vi "4 probe data v1.2.vi"() -> ()   [LabVIEW 2014]
uses:
  <vilib>/Analysis/baseanly.llb/Mean (DBL).vi
  <vilib>/MakerHub/LINX/Public/Peripherals/Analog/Analog Read 1 Chan.vi
  <instrlib>/Tektronix TDS 200 1000 2000 Series/Tektronix TDS 200 1000 2000 Series.lvlib
  <vilib>/MakerHub/LINX/LMH-LINX.lvlib
  <vilib>/Analysis/NI_AALBase.lvlib
panel:
  in  "Stop Button":bool
  out "Ard 4":dbl
  out "Ard 3":dbl
  out "Ard 2":dbl
  out "Ard 1":dbl
  out "Ard 0":dbl
  out "Data Ch4":string
  in  "Save File Ch4":path=path "C:/Users/Administrator/Documents/Device-characterization-setup/IV-Trace/Data/2015_xx_xx_xxxx_4-probe/2015_xx_xx_xxxx_Ch4_001.txt"
  out "Ard3-Osc4":cluster{"Y":dbl[], "Y":dbl[]}[](graph)
  out "Data Ch3":string
  in  "Save File Ch3":path=path "C:/Users/Administrator/Documents/Device-characterization-setup/IV-Trace/Data/2015_xx_xx_xxxx_4-probe/2015_xx_xx_xxxx_Ch3_001.txt"
  out "Ard2-Osc 3":cluster{"Y":dbl[], "Y":dbl[]}[](graph)
  out "Data Ch2":string
  in  "Save File Ch2":path=path "C:/Users/Administrator/Documents/Device-characterization-setup/IV-Trace/Data/2015_xx_xx_xxxx_4-probe/2015_xx_xx_xxxx_Ch2_001.txt"
  out "Ard1-Osc 2":cluster{"Y":dbl[], "Y":dbl[]}[](graph)
  out "Data Ch1":string
  in  "Save File Ch1":path=path "C:/Users/Administrator/Documents/Device-characterization-setup/IV-Trace/Data/2015_xx_xx_xxxx_4-probe/2015_xx_xx_xxxx_Ch1_001.txt"
  out "Ard0-Osc 1":cluster{"Y":dbl[], "Y":dbl[]}[](graph)
  out "Ch1":dbl
  out "Ch2":dbl
  out "Ch3":dbl
  out "Ch4":dbl
  out "Loop Rate (Hz)":u32
  out "Analog Data 4":dbl(graph)
  in  "AI Channel 4":u8=4
  in  "AI Channel 3":u8=3
  in  "AI Channel 2":u8=2
  in  "AI Channel 1":u8=1
  in  "AI Channel 0":u8
  in  "Serial Port":refnum<visa-resource-name>="COM6"
  in  "Channel 4 (3: Channel 4)":u16(ring)=3 items=["Channel 1", "Channel 2", "Channel 3", "Channel 4", "Math", "Reference A", "Reference B", "Reference C", "Reference D"]
  in  "Probe Attenuation 4 (0.1)":dbl=0.1
  in  "Vertical Coupling 4 (1: DC)":u16(ring)=1 items=["AC", "DC", "Ground"]
  in  "Channel 3 (2: Channel 3)":u16(ring)=2 items=["Channel 1", "Channel 2", "Channel 3", "Channel 4", "Math", "Reference A", "Reference B", "Reference C", "Reference D"]
  in  "Probe Attenuation 3 (0.1)":dbl=0.1
  in  "Vertical Coupling 3 (1: DC)":u16(ring)=1 items=["AC", "DC", "Ground"]
  in  "Channel 2 (1: Channel 2)":u16(ring)=1 items=["Channel 1", "Channel 2", "Channel 3", "Channel 4", "Math", "Reference A", "Reference B", "Reference C", "Reference D"]
  in  "Channel 1 (0: Channel 1)":u16(ring) items=["Channel 1", "Channel 2", "Channel 3", "Channel 4", "Math", "Reference A", "Reference B", "Reference C", "Reference D"]
  in  "Serial Configuration":T1={"Baud Rate"=9600, "Parity"=0, "Stop Bits"=10, "Flow Control"=2} {"Flow Control" items=["None", "XON/XOFF", "RTS/CTS", "XON/XOFF & RTS/CTS", "DTR/DSR", "XON/XOFF & DTR/DSR"]; "Stop Bits" items=["1.0"=10, "1.5"=15, "2.0"=20]; "Parity" items=["None", "Odd", "Even", "Mark", "Space"]; "Baud Rate" items=["300"=300, "600"=600, "1200"=1200, "2400"=2400, "4800"=4800, "9600"=9600, "19200"=19200]}
  in  "Probe Attenuation 2 (0.1)":dbl=0.1
  in  "Vertical Coupling 2 (1: DC)":u16(ring)=1 items=["AC", "DC", "Ground"]
  in  "Probe Attenuation 1 (0.1)":dbl=0.1
  in  "Vertical Coupling 1 (1: DC)":u16(ring)=1 items=["AC", "DC", "Ground"]
  in  "Timeout (10000 ms)":u32=500
  in  "VISA resource name":refnum<visa-resource-name>="USB0::0x0699::0x03A6::C044157::INSTR"
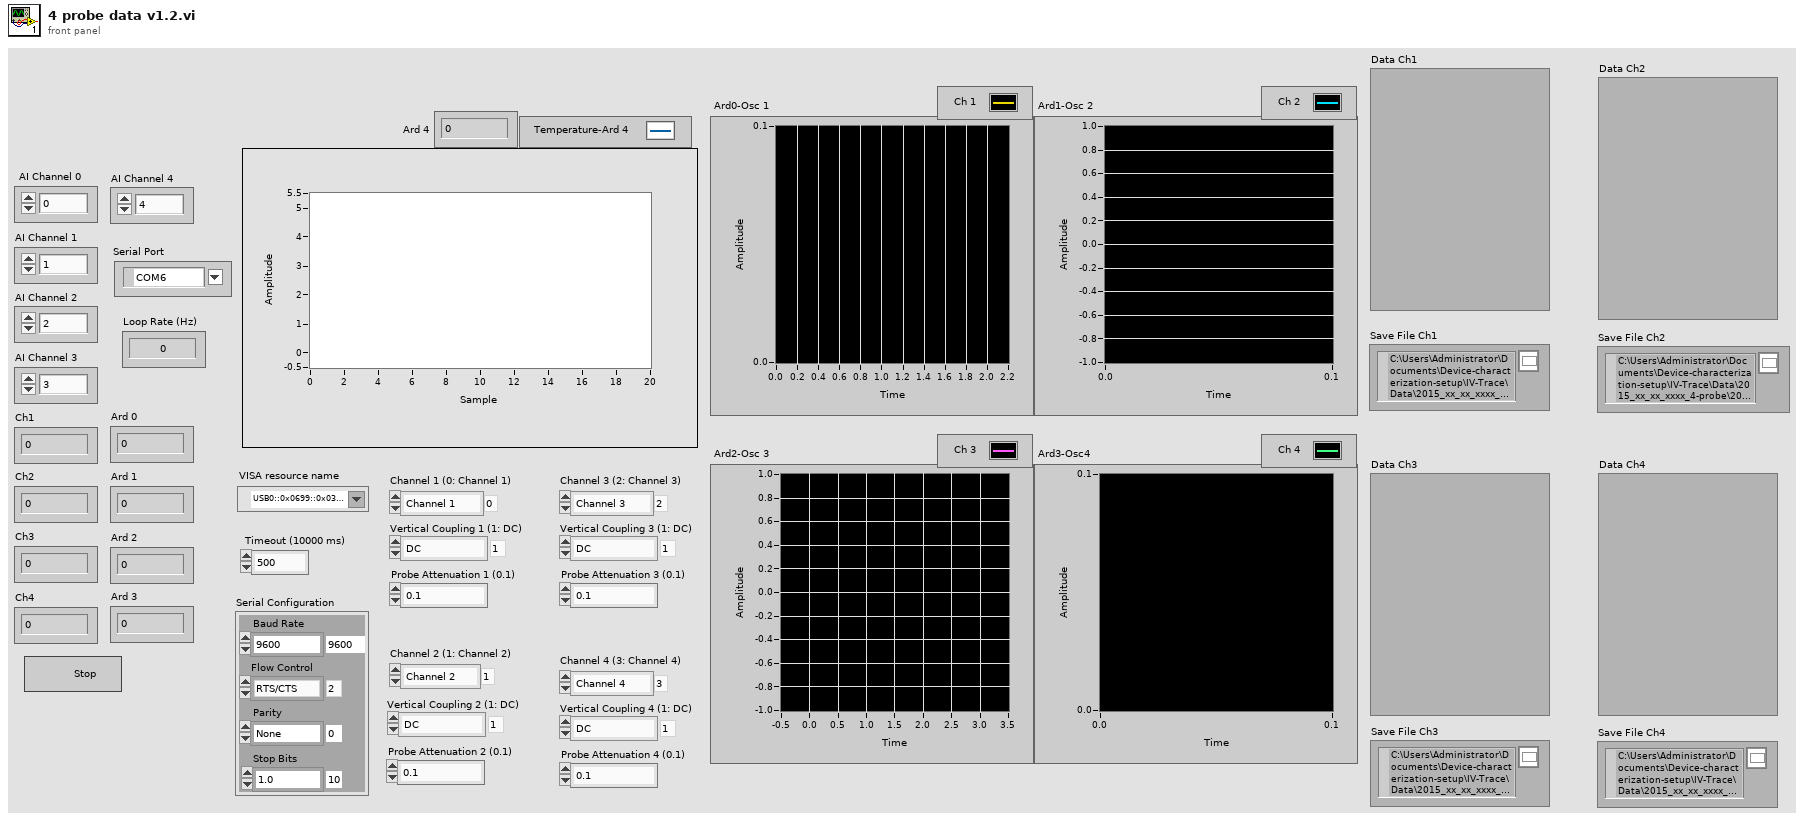
[diagram p1: front panel]
types:
  T1 = cluster{"Baud Rate":u32, "Parity":u16, "Stop Bits":u16, "Flow Control":u16}
  T2 = typedef "LMH-LINX.lvlib/LINX Ref.ctl" = cluster{"Platform":T3, "Interface":T4, "LINX Device Config":T5}
  T3 = typedef "LMH-LINX.lvlib/Platform.ctl" = enum16{"LINX", "myRIO"}
  T4 = typedef "LMH-LINX.lvlib/Interface.ctl" = enum16{"Serial", "TCP"}
  T5 = typedef "LMH-LINX.lvlib/Device.lvlib/LINX Device Config.ctl" = cluster{"Interface":T4, "COM Port":refnum<visa-resource-name>, "TCP Configuration":T6, "Device Family":u8, "Device ID":u8, "Device Name":string, "TCP Ref":refnum<k5>, "Channels":T7}
  T6 = typedef "LMH-LINX.lvlib/Device.lvlib/TCP Config.ctl" = cluster{"IP Address":string, "Port":u16}
  T7 = typedef "LMH-LINX.lvlib/Channels.ctl" = cluster{"DI":u8[], "DO":u8[], "AI":u8[], "AO":u8[], "PWM":u8[], "QE":u8[], "UART":u8[], "I2C 2":u8[], "SPI":u8[], "CAN":u8[], "Servo":u8[], "AI Ref (V)":dbl, "AO Ref (V)":dbl, "AO Resolution (Bits)":u8}
  T8 = enum16{"open", "replace", "create", "open or create", "replace or create", "replace or create with confirmation"}
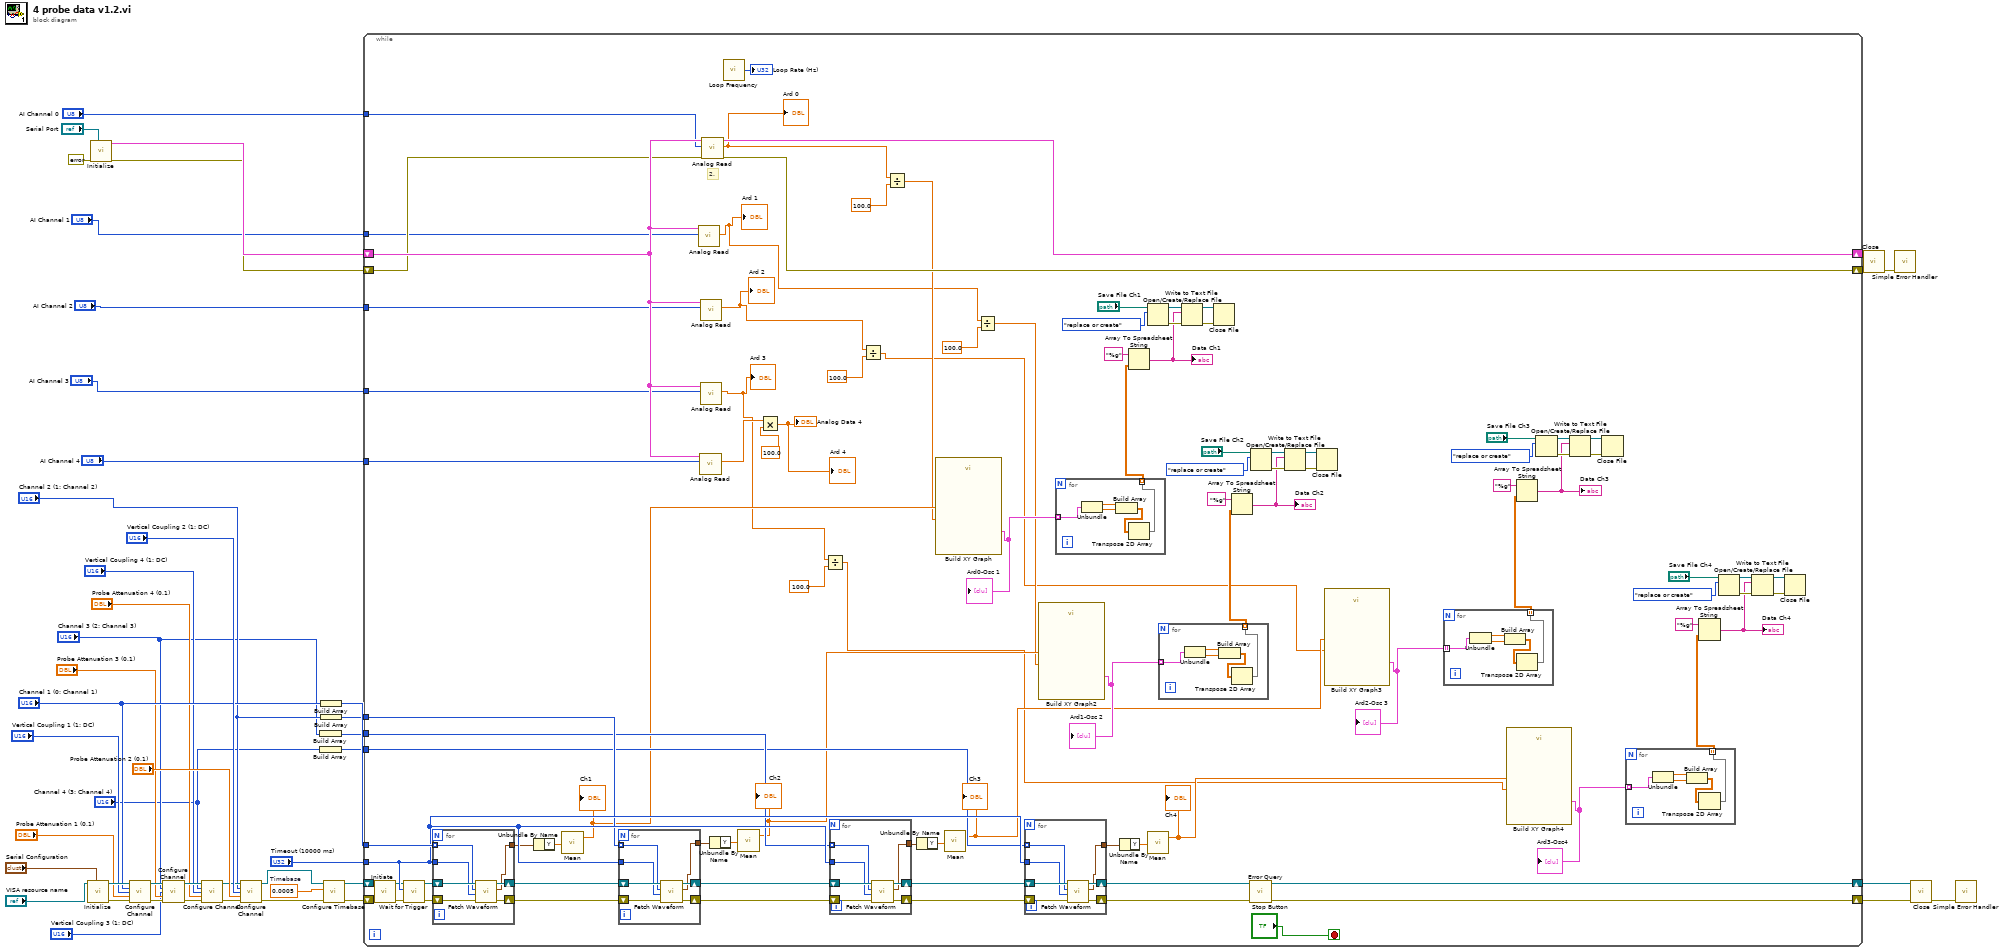
[diagram p0: block diagram]
diagram:
  w33 = 0.0005  # Timebase
  n1 = call <vilib>:"Initialize.vi"("Serial Configuration"="Serial Configuration", "VISA resource name"="VISA resource name") -> ("error out"=w42:errorcluster, "VISA resource name out"=w43:refnum<visa-resource-name>)  [unwired: 3 in, 5 out]
  n2 = call <vilib>:"Initialize.vi"("Serial Port"="Serial Port", "Error In"=errorcluster {"status"=FALSE, "code"=0, "source"=""}) -> ("Error Out"=w11:errorcluster, "LINX Ref"=w12:T2)  [unwired: 7 in, 1 out]
  n3 = call <instrlib>:"Configure Channel.vi"("VISA resource name"=w43, "Channel (0: Channel 1)"="Channel 1 (0: Channel 1)", "Vertical Coupling (1: DC)"="Vertical Coupling 1 (1: DC)", "Probe Attenuation (10: 10X)"="Probe Attenuation 1 (0.1)", "error in (no error)"=w42) -> ("VISA resource name out"=w28:refnum<visa-resource-name>, "error out"=w25:errorcluster)  [unwired: 4 in, 5 out]
  n4 = call <instrlib>:"Configure Channel.vi"("VISA resource name"=w28, "Channel (0: Channel 1)"="Channel 3 (2: Channel 3)", "Vertical Coupling (1: DC)"="Vertical Coupling 3 (1: DC)", "Probe Attenuation (10: 10X)"="Probe Attenuation 3 (0.1)", "error in (no error)"=w25) -> ("VISA resource name out"=w27:refnum<visa-resource-name>, "error out"=w24:errorcluster)  [unwired: 4 in, 5 out]
  n5 = call <instrlib>:"Configure Channel.vi"("VISA resource name"=w27, "Channel (0: Channel 1)"="Channel 4 (3: Channel 4)", "Vertical Coupling (1: DC)"="Vertical Coupling 4 (1: DC)", "Probe Attenuation (10: 10X)"="Probe Attenuation 4 (0.1)", "error in (no error)"=w24) -> ("VISA resource name out"=w26:refnum<visa-resource-name>, "error out"=w23:errorcluster)  [unwired: 4 in, 5 out]
  n6 = call <instrlib>:"Configure Channel.vi"("VISA resource name"=w26, "Channel (0: Channel 1)"="Channel 2 (1: Channel 2)", "Vertical Coupling (1: DC)"="Vertical Coupling 2 (1: DC)", "Probe Attenuation (10: 10X)"="Probe Attenuation 2 (0.1)", "error in (no error)"=w23) -> ("VISA resource name out"=w41:refnum<visa-resource-name>, "error out"=w40:errorcluster)  [unwired: 4 in, 5 out]
  n7 = Build Array("Channel 3 (2: Channel 3)") -> (w14:u16[])
  n8 = Build Array("Channel 4 (3: Channel 4)") -> (w13:u16[])
  n9 = Build Array("Channel 1 (0: Channel 1)") -> (w32:u16[])
  n10 = Build Array("Channel 2 (1: Channel 2)") -> (w17:u16[])
  n11 = call <instrlib>:"Configure Timebase.vi"("error in (no error)"=w40, "Timebase (0.0005 s)"=w33, "VISA resource name"=w41) -> ("error out"=w38:errorcluster, "VISA resource name out"=w39:refnum<visa-resource-name>)  [unwired: 1 in, 6 out]
  n12 = while {
    tunnel: w32 -> [w142]
    tunnel: "Timeout (10000 ms)" -> [w141]
    tunnel: w17 -> [w140]
    tunnel: w14 -> [w139]
    tunnel: w13 -> [w138]
    tunnel: "AI Channel 0" -> [w113]
    tunnel: "AI Channel 1" -> [w112]
    tunnel: "AI Channel 2" -> [w111]
    tunnel: "AI Channel 3" -> [w110]
    tunnel: "AI Channel 4" -> [w109]
    shift-right: [w146] -> w45
    shift-left: w39 -> [w144]
    shift-right: [w145] -> w44
    shift-left: w38 -> [w143]
    shift-right: [w115] -> w10
    shift-left: w12 -> [w117]
    shift-right: [w114] -> w9
    shift-left: w11 -> [w116]
    stop <- "Stop Button" stop-if-true
    # "2."
    n13 = call <instrlib>:"Initiate.vi"("error in (no error)"=w143, "VISA resource name"=w144) -> ("error out"=w134:errorcluster, "VISA resource name out"=w137:refnum<visa-resource-name>)  [unwired: 8 out]
    n14 = call <instrlib>:"Wait for Trigger.vi"("error in (no error)"=w134, "Timeout (10000 ms)"=w141, "VISA resource name"=w137) -> ("error out"=w135:errorcluster, "VISA resource name out"=w136:refnum<visa-resource-name>)  [unwired: 7 out]
    n15 = for {
      shift-right: [w193] -> w132
      shift-left: w135 -> [w191]
      tunnel: w142 -> [w189] mode=indexing
      tunnel: w141 -> [w190]
      shift-right: [w194] -> w133
      shift-left: w136 -> [w192]
      tunnel: [w188] -> w125
      n16 = call <instrlib>:"Fetch Waveform.vi"("error in (no error)"=w191, "Timeout (10000 ms)"=w190, "Source (0: Channel 1)"=w189, "VISA resource name"=w192) -> ("error out"=w193:errorcluster, "Waveform Data"=w188:waveform(dbl), "VISA resource name out"=w194:refnum<visa-resource-name>)  [unwired: 2 in, 3 out]
    }
    n17 = Unbundle By Name(w125) -> ("Y"=w124:dbl[])
    n18 = call-poly <vilib>:"Mean.vi"("X"=w124) -> ("mean"=w63:dbl)  [unwired: 1 out]
    "Ch1" <- w63
    n19 = for {
      shift-right: [w186] -> w126
      shift-left: w132 -> [w184]
      tunnel: w140 -> [w182] mode=indexing
      tunnel: w141 -> [w183]
      shift-right: [w187] -> w127
      shift-left: w133 -> [w185]
      tunnel: [w181] -> w121
      n20 = call <instrlib>:"Fetch Waveform.vi"("error in (no error)"=w184, "Timeout (10000 ms)"=w183, "Source (0: Channel 1)"=w182, "VISA resource name"=w185) -> ("error out"=w186:errorcluster, "Waveform Data"=w181:waveform(dbl), "VISA resource name out"=w187:refnum<visa-resource-name>)  [unwired: 2 in, 3 out]
    }
    n21 = call-poly <vilib>:"Analog Read.vi"("Analog Channel"=w112, "LINX Resource"=w117) -> ("AI Value"=w55:dbl)  [unwired: 6 in, 3 out]
    "Ard 1" <- w55
    n22 = call-poly <vilib>:"Analog Read.vi"("Analog Channel"=w109, "LINX Resource"=w117) -> ("AI Value"=w107:dbl)  [unwired: 6 in, 3 out]
    n23 = call-poly <vilib>:"Analog Read.vi"("Analog Channel"=w111, "LINX Resource"=w117) -> ("AI Value"=w52:dbl)  [unwired: 6 in, 3 out]
    "Ard 2" <- w52
    n24 = call-poly <vilib>:"Analog Read.vi"("Analog Channel"=w110, "LINX Resource"=w117) -> ("AI Value"=w49:dbl)  [unwired: 6 in, 3 out]
    "Ard 3" <- w49
    n25 = call-poly <vilib>:"Analog Read.vi"("Error In"=w116, "Analog Channel"=w113, "LINX Resource"=w117) -> ("Error Out"=w114:errorcluster, "AI Value"=w59:dbl, "LINX Resource"=w115:T2)  [unwired: 5 in, 1 out]
    "Ard 0" <- w59
    n26 = Unbundle By Name(w121) -> ("Y"=w120:dbl[])
    n27 = call <vilib>:"Loop Frequency.vi"() -> ("Loop Rate (Hz)"=→"Loop Rate (Hz)":u32)
    n28 = call-poly <vilib>:"Mean.vi"("X"=w120) -> ("mean"=w62:dbl)  [unwired: 1 out]
    "Ch2" <- w62
    n29 = Multiply(x=w107, y=100.0) -> (x*y=→"Analog Data 4" →"Ard 4":dbl)
    n30 = Divide(x=w49, y=100.0) -> (x/y=w48:dbl)
    n31 = for {
      shift-right: [w179] -> w130
      shift-left: w126 -> [w177]
      tunnel: w139 -> [w175] mode=indexing
      tunnel: w141 -> [w176]
      shift-right: [w180] -> w131
      shift-left: w127 -> [w178]
      tunnel: [w174] -> w122
      n32 = call <instrlib>:"Fetch Waveform.vi"("error in (no error)"=w177, "Timeout (10000 ms)"=w176, "Source (0: Channel 1)"=w175, "VISA resource name"=w178) -> ("error out"=w179:errorcluster, "Waveform Data"=w174:waveform(dbl), "VISA resource name out"=w180:refnum<visa-resource-name>)  [unwired: 2 in, 3 out]
    }
    n33 = Divide(x=w52, y=100.0) -> (x/y=w51:dbl)
    n34 = Divide(x=w59, y=100.0) -> (x/y=w58:dbl)
    n35 = Unbundle By Name(w122) -> ("Y"=w119:dbl[])
    n36 = call "Build XY Graph"("Y Input"=w58, "X Input"=w63) -> ("XY Graph"=w96:cluster{"Y":dbl[], "Y":dbl[]}[])  [unwired: 8 in, 1 out]
    "Ard0-Osc 1" <- w96
    n37 = call-poly <vilib>:"Mean.vi"("X"=w119) -> ("mean"=w61:dbl)  [unwired: 1 out]
    "Ch3" <- w61
    n38 = Divide(x=w55, y=100.0) -> (x/y=w54:dbl)
    n39 = for {
      shift-right: [w172] -> w128
      shift-left: w130 -> [w170]
      tunnel: w138 -> [w168] mode=indexing
      tunnel: w141 -> [w169]
      shift-right: [w173] -> w129
      shift-left: w131 -> [w171]
      tunnel: [w167] -> w123
      n40 = call <instrlib>:"Fetch Waveform.vi"("error in (no error)"=w170, "Timeout (10000 ms)"=w169, "Source (0: Channel 1)"=w168, "VISA resource name"=w171) -> ("error out"=w172:errorcluster, "Waveform Data"=w167:waveform(dbl), "VISA resource name out"=w173:refnum<visa-resource-name>)  [unwired: 2 in, 3 out]
    }
    n41 = call "Build XY Graph2"("Y Input"=w54, "X Input"=w62) -> ("XY Graph"=w86:cluster{"Y":dbl[], "Y":dbl[]}[])  [unwired: 8 in, 1 out]
    "Ard1-Osc 2" <- w86
    n42 = for {
      tunnel: w96 -> [w166] mode=indexing
      tunnel: [w162] -> w97 mode=indexing
      n43 = Unbundle(w166) -> ("Y"=w165:dbl[], "Y"=w164:dbl[])
      n44 = Build Array(w165, w164) -> (w163:dbl[][])
      n45 = Transpose 2D Array(2D array=w163) -> (transposed array=w162:dbl[][])
    }
    n46 = Unbundle By Name(w123) -> ("Y"=w118:dbl[])
    n47 = Array To Spreadsheet String(array=w97, 3:"%g" ("format string")) -> (spreadsheet string=w98:string)  [unwired: 1 in]
    "Data Ch1" <- w98
    n48 = Open/Create/Replace File(file path (use dialog)="Save File Ch1", operation (0:open)=T8."replace or create") -> (refnum out=w100:refnum<file>, error out=w105:errorcluster)  [unwired: 4 in, 1 out]
    n49 = call-poly <vilib>:"Mean.vi"("X"=w118) -> ("mean"=w60:dbl)  [unwired: 1 out]
    "Ch4" <- w60
    n50 = for {
      tunnel: w86 -> [w161] mode=indexing
      tunnel: [w157] -> w87 mode=indexing
      n51 = Unbundle(w161) -> ("Y"=w160:dbl[], "Y"=w159:dbl[])
      n52 = Build Array(w160, w159) -> (w158:dbl[][])
      n53 = Transpose 2D Array(2D array=w158) -> (transposed array=w157:dbl[][])
    }
    n54 = Write to Text File(file (use dialog)=w100, text=w98, error in=w105) -> (refnum out=w103:refnum<file>, error out=w104:errorcluster)  [unwired: 2 out]
    n55 = Close File(refnum=w103, error in=w104) -> ()  [unwired: 2 out]
    n56 = Array To Spreadsheet String(array=w87, 3:"%g" ("format string")) -> (spreadsheet string=w88:string)  [unwired: 1 in]
    "Data Ch2" <- w88
    n57 = call <instrlib>:"Error Query.vi"("error in (no error)"=w128, "VISA resource name"=w129) -> ("error out"=w145:errorcluster, "VISA resource name out"=w146:refnum<visa-resource-name>)  [unwired: 8 out]
    n58 = Open/Create/Replace File(file path (use dialog)="Save File Ch2", operation (0:open)=T8."replace or create") -> (refnum out=w90:refnum<file>, error out=w95:errorcluster)  [unwired: 4 in, 1 out]
    n59 = Write to Text File(file (use dialog)=w90, text=w88, error in=w95) -> (refnum out=w93:refnum<file>, error out=w94:errorcluster)  [unwired: 2 out]
    n60 = Close File(refnum=w93, error in=w94) -> ()  [unwired: 2 out]
    n61 = call "Build XY Graph3"("Y Input"=w51, "X Input"=w61) -> ("XY Graph"=w76:cluster{"Y":dbl[], "Y":dbl[]}[])  [unwired: 8 in, 1 out]
    "Ard2-Osc 3" <- w76
    n62 = for {
      tunnel: w76 -> [w156] mode=indexing
      tunnel: [w152] -> w77 mode=indexing
      n63 = Unbundle(w156) -> ("Y"=w155:dbl[], "Y"=w154:dbl[])
      n64 = Build Array(w155, w154) -> (w153:dbl[][])
      n65 = Transpose 2D Array(2D array=w153) -> (transposed array=w152:dbl[][])
    }
    n66 = call "Build XY Graph4"("Y Input"=w48, "X Input"=w60) -> ("XY Graph"=w66:cluster{"Y":dbl[], "Y":dbl[]}[])  [unwired: 8 in, 1 out]
    "Ard3-Osc4" <- w66
    n67 = Array To Spreadsheet String(array=w77, 3:"%g" ("format string")) -> (spreadsheet string=w78:string)  [unwired: 1 in]
    "Data Ch3" <- w78
    n68 = Open/Create/Replace File(file path (use dialog)="Save File Ch3", operation (0:open)=T8."replace or create") -> (refnum out=w80:refnum<file>, error out=w85:errorcluster)  [unwired: 4 in, 1 out]
    n69 = Write to Text File(file (use dialog)=w80, text=w78, error in=w85) -> (refnum out=w83:refnum<file>, error out=w84:errorcluster)  [unwired: 2 out]
    n70 = Close File(refnum=w83, error in=w84) -> ()  [unwired: 2 out]
    n71 = for {
      tunnel: w66 -> [w151] mode=indexing
      tunnel: [w147] -> w67 mode=indexing
      n72 = Unbundle(w151) -> ("Y"=w150:dbl[], "Y"=w149:dbl[])
      n73 = Build Array(w150, w149) -> (w148:dbl[][])
      n74 = Transpose 2D Array(2D array=w148) -> (transposed array=w147:dbl[][])
    }
    n75 = Array To Spreadsheet String(array=w67, 3:"%g" ("format string")) -> (spreadsheet string=w68:string)  [unwired: 1 in]
    "Data Ch4" <- w68
    n76 = Open/Create/Replace File(file path (use dialog)="Save File Ch4", operation (0:open)=T8."replace or create") -> (refnum out=w70:refnum<file>, error out=w75:errorcluster)  [unwired: 4 in, 1 out]
    n77 = Write to Text File(file (use dialog)=w70, text=w68, error in=w75) -> (refnum out=w73:refnum<file>, error out=w74:errorcluster)  [unwired: 2 out]
    n78 = Close File(refnum=w73, error in=w74) -> ()  [unwired: 2 out]
  }
  n79 = call <instrlib>:"Close.vi"("Error In"=w9, "LINX Resource"=w10) -> ("Error Out"=w7:errorcluster)  [unwired: 8 in, 1 out]
  n80 = call <vilib>:"Simple Error Handler.vi"("error in (no error)"=w7) -> ()  [unwired: 4 in, 5 out]
  n81 = call <instrlib>:"Close.vi"("error in (no error)"=w44, "VISA resource name"=w45) -> ("error out"=w46:errorcluster)  [unwired: 9 out]
  n82 = call <vilib>:"Simple Error Handler.vi"("error in (no error)"=w46) -> ()  [unwired: 1 in, 8 out]
